vi "Begin.vi"(8 "error in":errorcluster) -> (0 "error out":errorcluster)   [LabVIEW 2016]
doc: "Called before other user functions, this VI is expected to open initial I/O refnums, load in file data, and do all program initialization. Notice that the <B>error out</B> terminal is simply used for data flow. Wiring it to other structures or subVIs ensures that this VI runs first."
uses:
  <vilib>/Rock Robotics/SystemInterfaces/DIO/FPGA_DIOPWMChannel.ctl
  <vilib>/Rock Robotics/WPI/SafetyOutput/WPI_SafetyOutputConfigMenu.ctl
  <vilib>/Rock Robotics/WPI/DriverStation/WPI_DriverStationRobotMode2.ctl
  <vilib>/Rock Robotics/WPI/Joystick/WPI_JoystickDeviceEnum.ctl
  <vilib>/Rock Robotics/WPI/RobotDrive/WPI_RobotDriveOpen2MotorWithTalon.vi
  Robot Global Data.vi
  <vilib>/Rock Robotics/Network Tables/NT Write String Array.vi
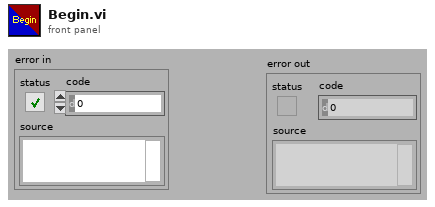
[diagram p1: front panel]
types:
  T1 = typedef "WPI_JoystickDeviceEnum.ctl" = enum16{"USB 0", "USB 1", "USB 2", "USB 3", "USB 4", "USB 5"}
  T2 = typedef "WPI_DriverStationRobotMode2.ctl" = enum16{"Autonomous Disabled", "Autonomous Enabled", "Teleop Disabled", "Teleop Enabled", "Disconnected", "Finish", "Test Disabled", "Test Enabled", "Emergency Stopped"}
  T3 = typedef "WPI_SafetyOutputConfigMenu.ctl" = enum16{"Enable", "Disable"}
  T4 = typedef "FPGA_DIOPWMChannel.ctl" = enum8{"PWM 0", "PWM 1", "PWM 2", "PWM 3", "PWM 4", "PWM 5", "PWM 6", "PWM 7", "PWM 8", "PWM 9", "PWM MXP 0", "PWM MXP 1", "PWM MXP 2", "PWM MXP 3", "PWM MXP 4", "PWM MXP 5", "PWM MXP 6", "PWM MXP 7", "PWM MXP 8", "PWM MXP 9", "Invalid"}
  T5 = typedef "WPI_JoystickDevRef.ctl" = cluster{"Device":T1}
  T6 = typedef "WPI_RobotDriveDevRef.ctl" = cluster{"DevStatus":errorcluster, "Motors[]":T7[], "Square Inputs":bool, "Max Output":dbl}
  T7 = typedef "WPI_MotorControlDeviceRef.ctl" = cluster{"DeviceStatus":errorcluster, "Type":T8, "PWM":cluster{"PWM Channel":T4, "DeadBand":T9}, "CAN":cluster{"Device Number":u8, "SetOutput VI Ref":variant, "GetOutput VI Ref":variant, "Enable VI Ref":variant, "Disable VI Ref":variant, "Data":variant}, "Invert":bool}
  T8 = typedef "WPI_MotorControlType.ctl" = enum16{"PWM", "CAN"}
  T9 = typedef "WPI_PWMDeadband.ctl" = cluster{"Name":string, "maxPositivePwm":i32, "minPositivePwm":i32, "centerPwm":i32, "maxNegativePwm":i32, "minNegativePwm":i32, "angularRange":u16}
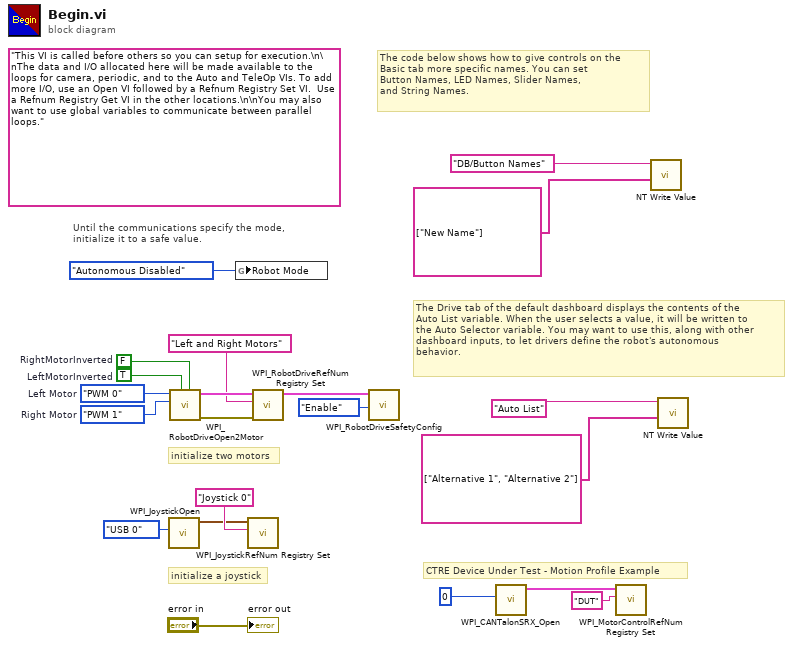
[diagram p0: block diagram]
diagram:
  (unwired) "This VI is called before others so you can setup for execution.\n\nThe data and I/O allocated here will be made available to the loops for camera, periodic, and to the Auto and TeleOp VIs. To add more I/O, use an Open VI followed by a Refnum Registry Set VI.  Use a Refnum Registry Get VI in the other locations.\n\nYou may also want to use global variables to communicate between parallel loops."
  w15 = FPGA_DIOPWMChannel."PWM 1"  # Right Motor
  w16 = FPGA_DIOPWMChannel."PWM 0"  # Left Motor
  w20 = TRUE  # LeftMotorInverted
  w21 = FALSE  # RightMotorInverted
  # "CTRE Device Under Test - Motion Profile Example"
  # "The Drive tab of the default dashboard displays the contents of the\nAuto List variable. When the user selects a value, it will be written to\nthe Auto Selector variable. You may want to use this, along with other\ndashboard inputs, to let drivers define the robot's autonomous\nbehavior."
  # "The code below shows how to give controls on the\nBasic tab more specific names. You can set\nButton Names, LED Names, Slider Names,\nand String Names."
  # "initialize a joystick"
  # "Until the communications specify the mode,\ninitialize it to a safe value."
  # "initialize two motors"
  n1 = call <vilib>:"WPI_JoystickOpen.vi"("JoystickDevice"=WPI_JoystickDeviceEnum."USB 0") -> ("JoystickDevRef"=w10:T5)  [unwired: 10 in]
  n2 = call-poly <vilib>:"WPI_RobotDriveOpen2Motor.vi"("Right Motor Inverted"=w21, "Left Motor Inverted"=w20, "Right Motor"=w15, "Left Motor"=w16) -> ("error out"=w17:errorcluster, "RobotDriveDevRef"=w19:T6)  [unwired: 1 in, 5 out]
  n3 = global write "Robot Global Data.vi" "Robot Mode"(WPI_DriverStationRobotMode2."Autonomous Disabled" ("Robot Mode")) -> ()
  n4 = call <vilib>:"WPI_JoystickRefNum Registry Set.vi"("refnum name"="Joystick 0", "JoystickDevRef"=w10) -> ()  [unwired: 8 in, 2 out]
  n5 = call <vilib>:"WPI_RobotDriveRefNum Registry Set.vi"("error in (no error)"=w17, "refnum name"="Left and Right Motors", "RobotDriveDevRef"=w19) -> ("RobotDriveDevRef"=w14:T6)  [unwired: 1 in, 7 out]
  n6 = call <vilib>:"WPI_RobotDriveSafetyConfig.vi"("mode"=WPI_SafetyOutputConfigMenu."Enable", "RobotDriveDevRef"=w14) -> ()  [unwired: 8 in, 2 out]
  n7 = call <vilib>:"WPI_CANTalonSRX_Open.vi"("Device Number"=u8 0) -> ("CAN Talon SRX Ref"=w3:T7)  [unwired: 9 in, 1 out]
  n8 = call <vilib>:"WPI_MotorControlRefNum Registry Set.vi"("refnum name"="DUT", "MotorControlDevRef"=w3) -> ()  [unwired: 8 in, 2 out]
  n9 = call-poly <vilib>:"NT Write Value.vi"("String Array"=string[] ["New Name"], "Name"="DB/Button Names") -> ()  [unwired: 9 in, 1 out]
  n10 = call-poly <vilib>:"NT Write Value.vi"("String Array"=string[] ["Alternative 1", "Alternative 2"], "Name"="Auto List") -> ()  [unwired: 9 in, 1 out]
  "error out" <- "error in"
